vi "Coord window-Bring selection in view.vi"(8 "error in (no error)":errorcluster, 10 "Index of selected row":i32, 11 "MulticolumnListbox in":refnum<vi>) -> (0 "error out":errorcluster, 3 "MulticolumnListbox out":refnum<vi>)   [LabVIEW 2013]
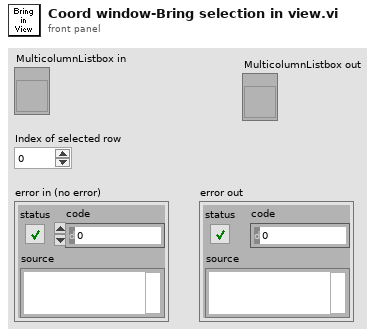
[diagram p1: front panel]
types:
  T1 = typedef "LVRowAndColumnUnsignedTypeDef.ctl" = cluster{"Row":u32, "Column":u32}
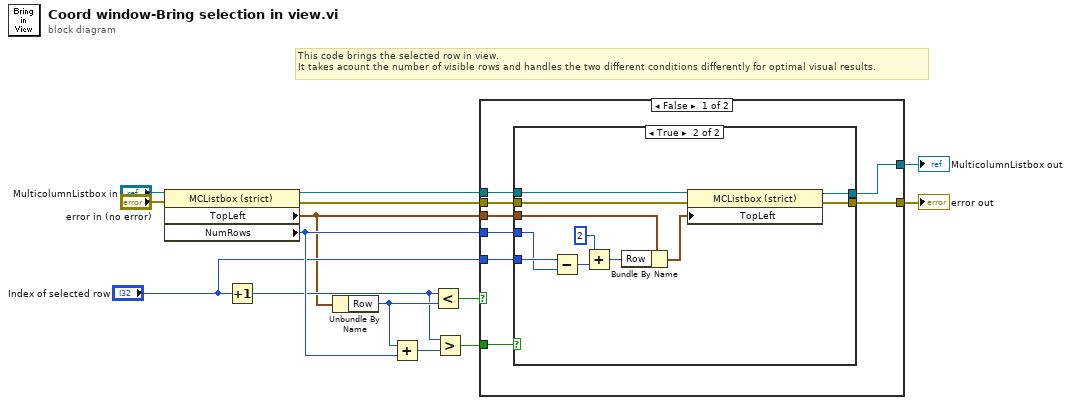
[diagram p0: block diagram]
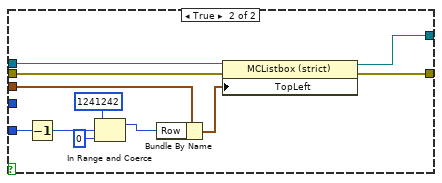
[diagram p3: hidden frame]
diagram:
  # "This code brings the selected row in view.\nIt takes acount the number of visible rows and handles the two different conditions differently for optimal visual results."
  n1 = property on="Property Node" class="MCListbox (strict)"(reference="MulticolumnListbox in", error in="error in (no error)") -> (reference out=w2:refnum<vi>, error out=w13:errorcluster, "TopLeft"=w5:T1, "NumRows"=w12:u32)
  n2 = Increment(x="Index of selected row") -> (x+1=w8:i32)
  n3 = Unbundle By Name(w5) -> ("Row"=w10:u32)
  n4 = Add(x=w10, y=w12) -> (x+y=w11:u32)
  n5 = Less?(x=w8, y=w10) -> (x < y?=w7:bool)
  n6 = Greater?(x=w8, y=w11) -> (0:w9:bool)
  n7 = case shown="False" w7 {
    tunnel: w2 -> [w22 w46]
    tunnel: w5 -> [w21 w45]
    tunnel: "Index of selected row" -> [w19 w43]
    tunnel: w9 -> [w20 _]
    tunnel: w12 -> [w18 _]
    tunnel: w13 -> [w17 w38]
    tunnel: [w16 w37] -> w14
    tunnel: [w15 w36] -> w1
    frame False {
      n8 = case shown="True" w20 {
        tunnel: w22 -> [w23 w35]
        tunnel: w21 -> [_ w34]
        tunnel: w19 -> [_ w32]
        tunnel: w18 -> [_ w31]
        tunnel: w17 -> [w24 w27]
        tunnel: [w24 w26] -> w16
        tunnel: [w23 w25] -> w15
        frame False {
        }
        frame True {
          n9 = Subtract(x=w32, y=w31) -> (x-y=w30:u32)
          n10 = Add(x=u32 2, y=w30) -> (x+y=w29:u32)
          n11 = Bundle By Name(cluster=w34, "Row"=w29) -> (w33:T1)
          n12 = property class="MCListbox (strict)"(reference=w35, error in=w27, "TopLeft"=w33) -> (reference out=w25:refnum<vi>, error out=w26:errorcluster)
        }
      }
    }
    frame True {
      n13 = Decrement(x=w43) -> (x-1=w42:i32)
      n14 = In Range and Coerce(upper limit=1241242, x=w42, lower limit=0) -> (coerced(x)=w41:i32)  [unwired: 1 out]
      n15 = Bundle By Name(cluster=w45, "Row"=w41) -> (w44:T1)
      n16 = property class="MCListbox (strict)"(reference=w46, error in=w38, "TopLeft"=w44) -> (reference out=w36:refnum<vi>, error out=w37:errorcluster)
    }
  }
  "error out" <- w14
  "MulticolumnListbox out" <- w1
